vi "Post Process Data Averaging.vi"(0 "pInputImage":i32, 1 "iAveragingFilterMode":i32, 2 "iWidth":i32, 3 "iAveragingFactor":i32, 5 "pOutputImage":i32, 7 "iOutputBufferSize":i32, 9 "iNumImages":i32, 11 "error in (no error)":errorcluster, 12 "iHeight":i32, 13 "iFrameCount":i32) -> (4 "pInputImage out":i32, 6 "pOutputImage out":i32, 8 "function return":u32, 15 "error out":errorcluster)   [LabVIEW 2014, in "atmcd32d.lvlib"]
doc: "unsigned int WINAPI PostProcessDataAveraging(at_32 * pInputImage, at_32 * pOutputImage, int iOutputBufferSize, int iNumImages, int iAveragingFilterMode, int iHeight, int iWidth, int iFrameCount, int iAveragingFactor);"
uses:
  atmcd32d.lvlib
  atmcd32d.dll
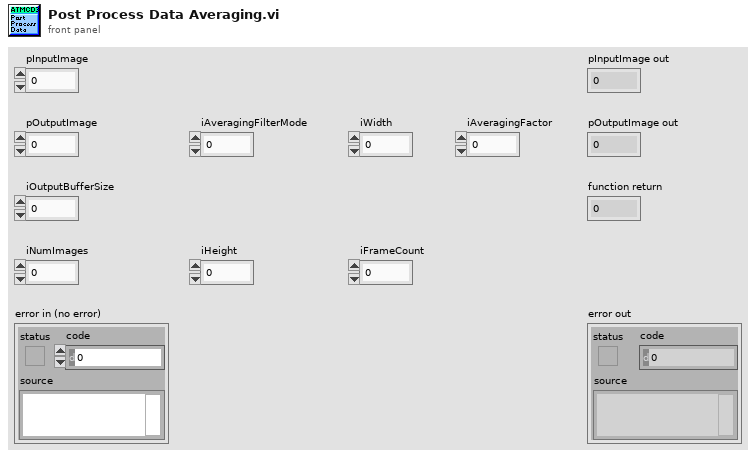
[diagram p1: front panel]
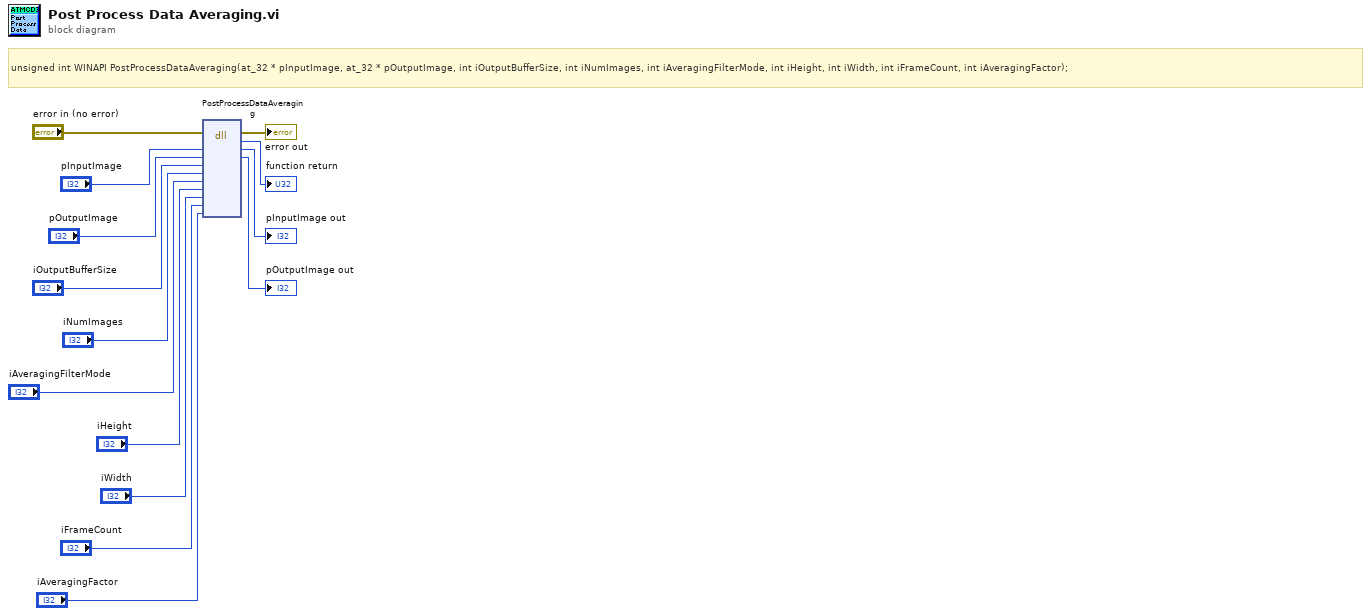
[diagram p0: block diagram]
diagram:
  # "unsigned int WINAPI PostProcessDataAveraging(at_32 * pInputImage, at_32 * pOutputImage, int iOutputBufferSize, int iNumImages, int iAveragingFilterMode, int iHeight, int iWidth, int iFrameCount, int iAveragingFactor);"
  n1 = dll-call lib="C:/Users/Bakir/Documents/Lambda2-Testing/lib/Andorlib/atmcd32d.*" fn="PostProcessDataAveraging"(error in="error in (no error)", "pInputImage"="pInputImage", "pOutputImage"="pOutputImage", "iOutputBufferSize"="iOutputBufferSize", "iNumImages"="iNumImages", "iAveragingFilterMode"="iAveragingFilterMode", "iHeight"="iHeight", "iWidth"="iWidth", "iFrameCount"="iFrameCount", "iAveragingFactor"="iAveragingFactor") -> (error out=→"error out":errorcluster, →"function return":u32, "pInputImage"=→"pInputImage out":i32, "pOutputImage"=→"pOutputImage out":i32)  [unwired: 9 in, 1 out]
